vi "SetValue.vi"(8 "error in":errorcluster, 10 "Value":string, 11 "StringMeasure in":refnum<class "StringMeasure.lvclass">) -> (0 "error out":errorcluster, 3 "StringMeasure out":refnum<class "StringMeasure.lvclass">)   [LabVIEW 2021, in "ProligentXMLGenerator.lvlib" / "StringMeasure.lvclass"]
doc: "Defines the value acquired by the measure."
uses:
  StringMeasure.lvclass
  StringMeasure.lvclass/StringMeasure.ctl
  Base/String_4000/String_4000.lvclass
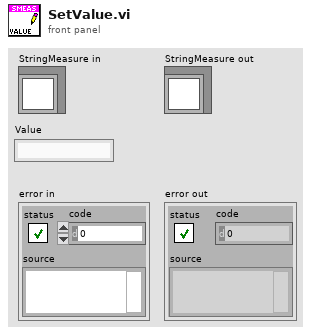
[diagram p1: front panel]
types:
  T1 = typedef "ProligentXMLGenerator.lvlib/StringMeasure.lvclass/Data.ctl" = cluster{"Value":refnum<class "String_4000.lvclass">}
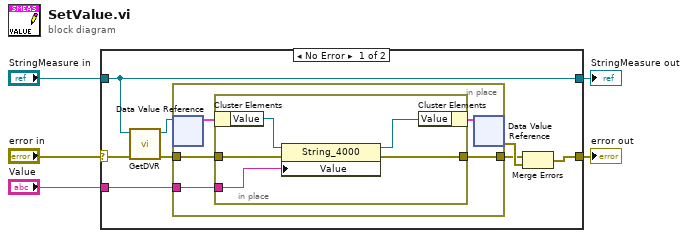
[diagram p0: block diagram]
diagram:
  n1 = case shown="No Error" "error in" {
    selector: "error in" -> [w11 w24]
    tunnel: "StringMeasure in" -> [w12 w25]
    tunnel: [w13 w24] -> w3
    tunnel: "Value" -> [w6 _]
    tunnel: [w12 w25] -> w1
    frame No Error {
      n2 = call "GetDVR.vi"("error in"=w11, "StringMeasure"=w12) -> ("error out"=w9:errorcluster, "DVRReference"=w10:refnum<data-value>)  [unwired: 8 in]
      n3 = in-place "In Place Element Structure" {
        in-place-border: w6 -> [w17]
        in-place-border: w9 -> [w18]
        in-place-border: [w16] -> w7
        n4 = in-place-dvr #1(w10) -> (w15:T1)  [unwired: 1 out]
        n5 = in-place {
          in-place-border: w18 -> [w23]
          in-place-border: w17 -> [w22]
          in-place-border: [w21] -> w16
          n6 = in-place-cluster #2(w15) -> ("Value"=w20:refnum<class "String_4000.lvclass">)
          n7 = property class="String_4000"(reference=w20, error in=w23, "Value"=w22) -> (reference out=w19:refnum<class "String_4000.lvclass">, error out=w21:errorcluster)
          n8 = in-place-cluster #2("Value"=w19) -> (w14:T1)
        }
        n9 = in-place-dvr #1(w14) -> (w8:errorcluster)  [unwired: 1 out]
      }
      n10 = Merge Errors(w7, w8) -> (w13:errorcluster)
    }
    frame Error {
    }
  }
  "error out" <- w3
  "StringMeasure out" <- w1
